vi "Create.vi"   [LabVIEW 2018, in "Toolkit.lvlib" / "Agent Identity.lvclass"]
doc: "Create an Agent Identity object. This allocates memory. To avoid memory leaks and possibly running out of memory (OOM) on resource constrained hardware, the memory allocated by this VI should be deallocated, or freed, using the Destroy VI.\n\nAn Agent Identity is a SSH username, public/private key, and passphrase/password for a remote server stored in a SSH agent application."
uses:
  Agent Identity.lvclass
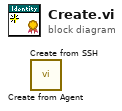
[diagram p0: block diagram]
diagram:
  n1 = call "Create from Agent.vi"() -> ()  [unwired: 9 in, 3 out]
  n2 = call "Create from SSH.vi"() -> ()  [unwired: 10 in, 2 out]
